vi "Example 6 - Get Abstract Class.vi"() -> ()   [LabVIEW 2021]
uses:
  Omni-Bus/Omni_Bus.lvclass
  Omni-Bus/Support/Broad Types.ctl
  Local Bus/Local Bus.lvclass
  C:/Users/Tim/Documents/GitHub/Omni-Bus/Source/Omni-Bus/Bus Access/Bus_Access.lvclass
  <vilib>/Utility/Data Type/Type Definitions/Data Type.ctl
  <vilib>/TSA/Abstract Data Classes/Abs_Types/Type/Abs_Type.lvclass/Abs_Type.ctl
  Omni-Bus/Omni_Bus.lvclass/Omni_Bus.ctl
  <vilib>/TSA/Abstract Data Classes/Abs_Types/Boolean/Static Write.vi
  <vilib>/TSA/Abstract Data Classes/Abs_Types/Boolean/Static Read.vi
  Omni-Bus/Support/FindVar.vi
  <vilib>/Utility/error.llb/Clear Errors.vi
  Omni-Bus/Properties/Read Var Map.vi
  <vilib>/TSA/Abstract Data Classes/Abs_Types/Type/Properties/Read Tag.vi
  <vilib>/TSA/Abstract Data Classes/Abs_Types/String/Abs_String.lvclass
  C:/Program Files (x86)/National Instruments/LabVIEW 2021/vi.lib/TSA/Abstract Data Classes/Abs_Types/Type/Abs_Type.lvclass
  <vilib>/TSA/Abstract Data Classes/Abs_Types/Value/Abs_Value.lvclass
  <vilib>/TSA/Abstract Data Classes/Abs_Types/U16 Integer/Abs_U16 Integer.lvclass
  <vilib>/TSA/Abstract Data Classes/Abs_Types/Boolean/Abs_Boolean.lvclass
  <vilib>/TSA/Abstract Data Classes/Abs_Types/Double Float/Abs_Double Float.lvclass
  Omni-Bus/Support/Check For Read Only Error.vi
  Omni-Bus/Support/Incorrect Tag String Error.vi
  <vilib>/TSA/Abstract Data Classes/Abs_Types/Type/Abs_Type.lvclass
  <vilib>/Utility/Data Type/NI_Data Type.lvlib
  C:/Users/Tim/Documents/GitHub/Omni-Bus/Source/Local Bus/Local Bus.lvclass
  Omni-Bus/Support/Get/Get String.vi
  <vilib>/TSA/Abstract Data Classes/Abs_Types/String/Static Write.vi
  <vilib>/TSA/Abstract Data Classes/Abs_Types/String/Static Read.vi
  Omni-Bus/Support/Get/Get U16.vi
  <vilib>/TSA/Abstract Data Classes/Abs_Types/U16 Integer/Static Write.vi
  <vilib>/TSA/Abstract Data Classes/Abs_Types/U16 Integer/Static Read.vi
  Omni-Bus/Support/Get/Get Boolean.vi
  Omni-Bus/Support/Get/Get DBL.vi
  <vilib>/TSA/Abstract Data Classes/Abs_Types/Double Float/Static Write.vi
  <vilib>/TSA/Abstract Data Classes/Abs_Types/Double Float/Static Read.vi
panel:
  out "DBL":dbl
  in  "DBL":dbl
  out "Boolean 2":bool
  in  "Boolean":bool
  out "U16":u16
  in  "U16":u16
  out "String":string
  in  "String":string
  in  "stop":bool
  out "All Tags":string[](array[string])
  # "The Get methods are responsible for the Tag to class mapping.\nSeparating the Get methods from the read and write methods adds \nimproves execution efficiency"
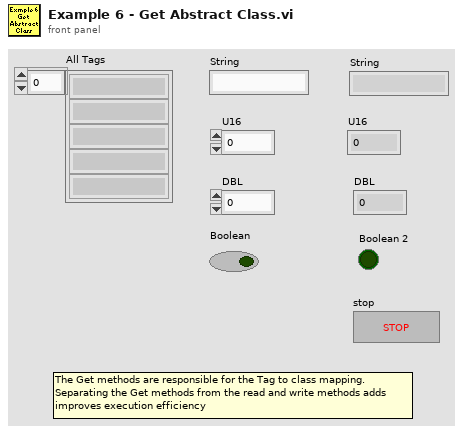
[diagram p1: front panel]
types:
  T1 = typedef "NI_Data Type.lvlib/Data Type.ctl" = enum8{"Invalid Type", "Void", "I8", "I16", "I32", "I64", "U8", "U16", "U32", "U64", "Single Float", "Double Float", "Extended Float", "Single Complex", "Double Complex", "Extended Complex", "Enum U8", "Enum U16", "Enum U32", "Enum U64", "Single Float With Unit", "Double Float With Unit", "Extended Float With Unit", "Single Complex with Unit", "Double Complex with Unit", "Extended Complex with Unit", "Boolean", "String", "Path", "Picture", "Tag", "Array", "Cluster", "Variant", "LV Variant", "Waveform", "Timestamp", "Digital Waveform", "Digital Data", "ExpressData", "Refnum", "External Data", "VI", "Poly VI", "LabVIEW Class Instance", "Fixed Point", "Set Collection", "Map Collection"}
  T2 = typedef "Omni_Bus.lvclass/Broad Types.ctl" = enum16{"All Tags", "NI Specific Type", "Boolean", "String", "Numeric", "Float", "Integer", "Collection", "All Value Types", "Non Value Types"}
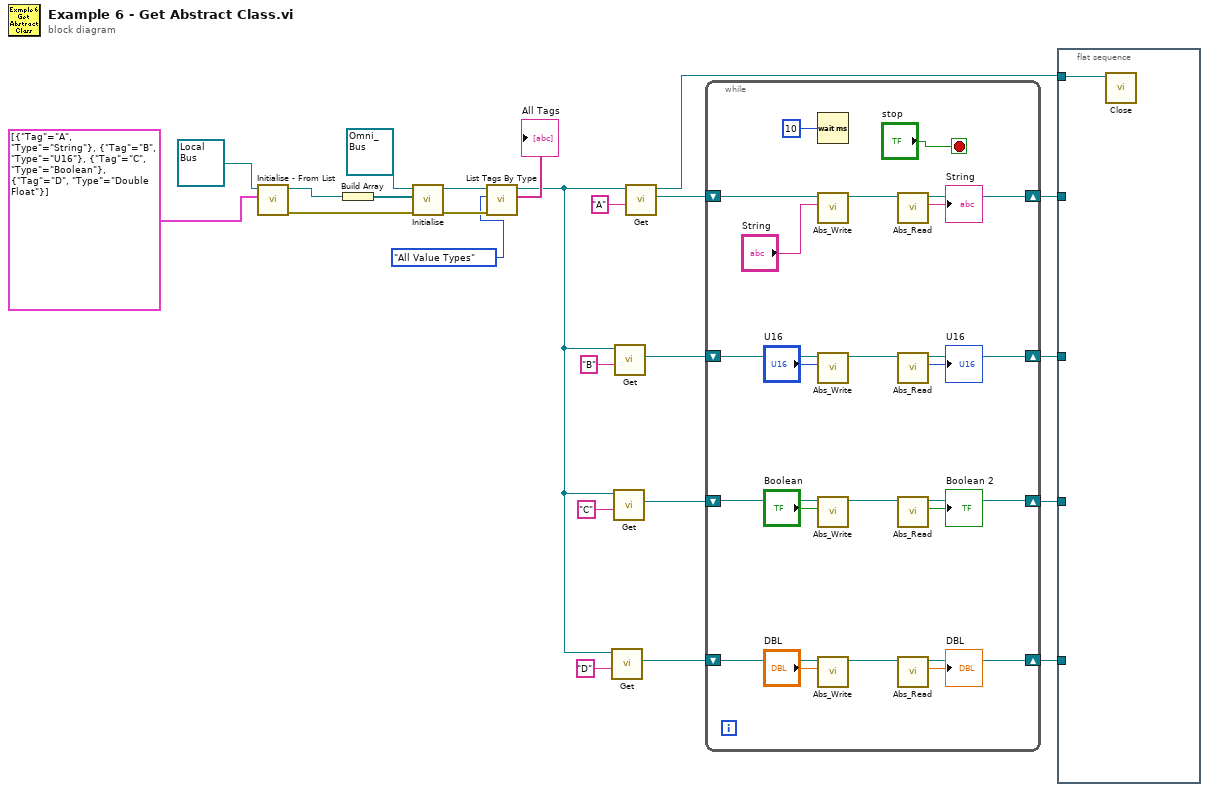
[diagram p0: block diagram]
diagram:
  n1 = call "Initialise - From List.vi"("Tag List"=cluster{"Tag":string, "Type":T1}[] [{"Tag"="A", "Type"=enum."String"}, {"Tag"="B", "Type"=enum."U16"}, {"Tag"="C", "Type"=enum."Boolean"}, {"Tag"="D", "Type"=enum."Double Float"}], "Local Bus in"=refnum<class "Local Bus.lvclass"> refnum ("Local Bus.lvclass")) -> ("error out"=w18:errorcluster, "Local Bus out"=w17:refnum<class "Local Bus.lvclass">)  [unwired: 8 in]
  n2 = Build Array(w17) -> (w23:refnum<class "Local Bus.lvclass">[])
  n3 = call-dynamic "Initialise.vi"("error in (no error)"=w18, "Bus Access"=w23, "Var Bus in"=refnum<class "Omni_Bus.lvclass"> refnum) -> ("error out"=w21:errorcluster, "Var Bus out"=w22:refnum<class "Omni_Bus.lvclass">)  [unwired: 7 in]
  n4 = call "List Tags By Type.vi"("error in (no error)"=w21, "Broad Types"=Broad_Types."All Value Types", "Var Bus in"=w22) -> ("Tags"=→"All Tags":string[], "Var Bus out"=w6:refnum<class "Omni_Bus.lvclass">)  [unwired: 5 in, 2 out]
  n5 = call-poly "Get.vi"("Tag"="D", "Var Bus in"=w6) -> ("Value Out"=w7:refnum<class "Abs_Double Float.lvclass">)  [unwired: 6 in, 3 out]
  n6 = call-poly "Get.vi"("Tag"="C", "Var Bus in"=w6) -> ("Value Out"=w8:refnum<class "Abs_Boolean.lvclass">)  [unwired: 6 in, 3 out]
  n7 = call-poly "Get.vi"("Tag"="B", "Var Bus in"=w6) -> ("Value Out"=w5:refnum<class "Abs_U16 Integer.lvclass">)  [unwired: 6 in, 3 out]
  n8 = call-poly "Get.vi"("Tag"="A", "Var Bus in"=w6) -> ("Value Out"=w14:refnum<class "Abs_String.lvclass">, "Var Bus out"=w12:refnum<class "Omni_Bus.lvclass">)  [unwired: 6 in, 2 out]
  n9 = while {
    shift-right: [w34] -> w9
    shift-left: w5 -> [w46]
    shift-right: [w35] -> w10
    shift-left: w8 -> [w44]
    shift-right: [w32] -> w11
    shift-left: w7 -> [w43]
    shift-right: [w39] -> w13
    shift-left: w14 -> [w42]
    stop <- "stop" stop-if-true
    n10 = Wait (ms)(milliseconds to wait=u32 10) -> ()  [unwired: 1 out]
    n11 = call-poly <vilib>:"Abs_Write.vi"("String"="String", "Abs_String in"=w42) -> ("Abs_String out"=w40:refnum<class "Abs_String.lvclass">)  [unwired: 8 in, 1 out]
    n12 = call-poly <vilib>:"Abs_Write.vi"("Value"="U16", "Abs_U16 Integer in"=w46) -> ("Abs_U16 Integer out"=w37:refnum<class "Abs_U16 Integer.lvclass">)  [unwired: 8 in, 1 out]
    n13 = call-poly <vilib>:"Abs_Write.vi"("Boolean"="Boolean", "Abs_Boolean in"=w44) -> ("Abs_Boolean out"=w36:refnum<class "Abs_Boolean.lvclass">)  [unwired: 8 in, 1 out]
    n14 = call-poly <vilib>:"Abs_Write.vi"("Value"="DBL", "Abs_Double Float in"=w43) -> ("Abs_Double Float out"=w33:refnum<class "Abs_Double Float.lvclass">)  [unwired: 8 in, 1 out]
    n15 = call-poly <vilib>:"Abs_Read.vi"("Abs_String in"=w40) -> ("String"=→"String":string, "Abs_String out"=w39:refnum<class "Abs_String.lvclass">)  [unwired: 8 in, 1 out]
    n16 = call-poly <vilib>:"Abs_Read.vi"("Abs_U16 Integer in"=w37) -> ("Value"=→"U16":u16, "Abs_U16 Integer out"=w34:refnum<class "Abs_U16 Integer.lvclass">)  [unwired: 8 in, 1 out]
    n17 = call-poly <vilib>:"Abs_Read.vi"("Abs_Boolean in"=w36) -> ("Boolean"=→"Boolean 2":bool, "Abs_Boolean out"=w35:refnum<class "Abs_Boolean.lvclass">)  [unwired: 8 in, 1 out]
    n18 = call-poly <vilib>:"Abs_Read.vi"("Abs_Double Float in"=w33) -> ("Value"=→"DBL":dbl, "Abs_Double Float out"=w32:refnum<class "Abs_Double Float.lvclass">)  [unwired: 8 in, 1 out]
  }
  n19 = flat-sequence {
    tunnel: w13 -> [_]
    tunnel: w12 -> [w47]
    tunnel: w11 -> [_]
    tunnel: w10 -> [_]
    tunnel: w9 -> [_]
    frame #0 {
      n20 = call-dynamic "Close.vi"("Data in"=w47) -> ()  [unwired: 9 in, 2 out]
    }
  }
